vi "Close Variable Connections.vi"(11 "Variable References":T1) -> ()   [LabVIEW 2017]
uses:
  controls/Variable References.ctl
  controls/Control State.ctl
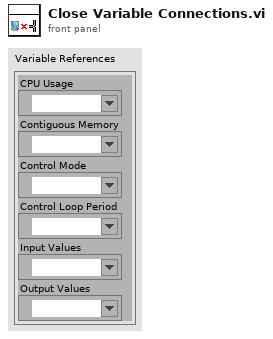
[diagram p1: front panel]
types:
  T1 = typedef "Variable References.ctl" = cluster{"CPU Usage":refnum<k21>, "Contiguous Memory":refnum<k21>, "Control Mode":refnum<k21>, "Control Loop Period":refnum<k21>, "Input Values":refnum<k21>, "Output Values":refnum<k21>}
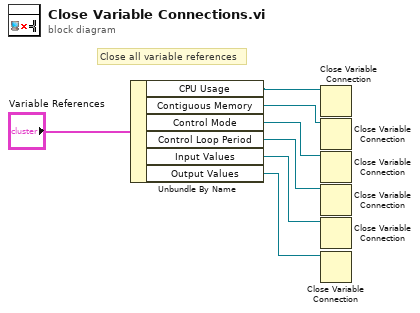
[diagram p0: block diagram]
diagram:
  # "Close all variable references"
  n1 = Unbundle By Name("Variable References") -> ("CPU Usage"=w4:refnum<k21>, "Contiguous Memory"=w5:refnum<k21>, "Control Mode"=w6:refnum<k21>, "Control Loop Period"=w7:refnum<k21>, "Input Values"=w2:refnum<k21>, "Output Values"=w1:refnum<k21>)
  n2 = Close Variable Connection(11:w4) -> ()  [unwired: 1 in, 1 out]
  n3 = Close Variable Connection(11:w5) -> ()  [unwired: 1 in, 1 out]
  n4 = Close Variable Connection(11:w6) -> ()  [unwired: 1 in, 1 out]
  n5 = Close Variable Connection(11:w7) -> ()  [unwired: 1 in, 1 out]
  n6 = Close Variable Connection(11:w2) -> ()  [unwired: 1 in, 1 out]
  n7 = Close Variable Connection(11:w1) -> ()  [unwired: 1 in, 1 out]
